vi "Generate Mass Spreadsheet Data.vi"() -> ()   [LabVIEW 2010]
uses:
  Controls/Spreadsheet Commands.ctl
  <vilib>/measure/NI_MABase.lvlib
panel:
  out "F-format string":string[][](array[string])
  in  "Channel Names":string[](array[string])
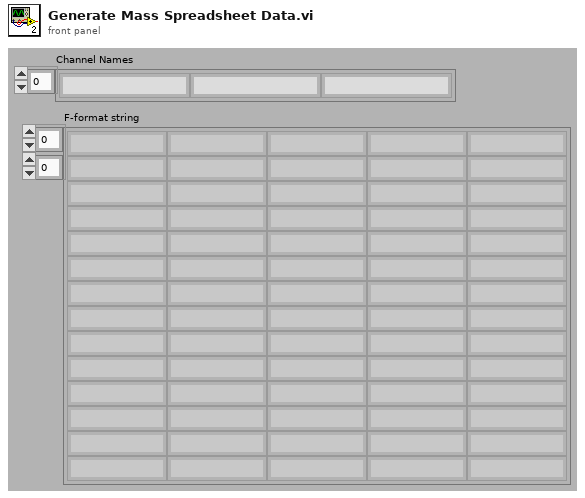
[diagram p1: front panel]
types:
  T1 = typedef "Spreadsheet Commands.ctl" = enum16{"Init", "Clear", "Add", "Mass Add", "Delete Row", "Format Colors", "Stop"}
  T2 = enum16{"Sine Wave", "Triangle Wave", "Square Wave", "Sawtooth Wave"}
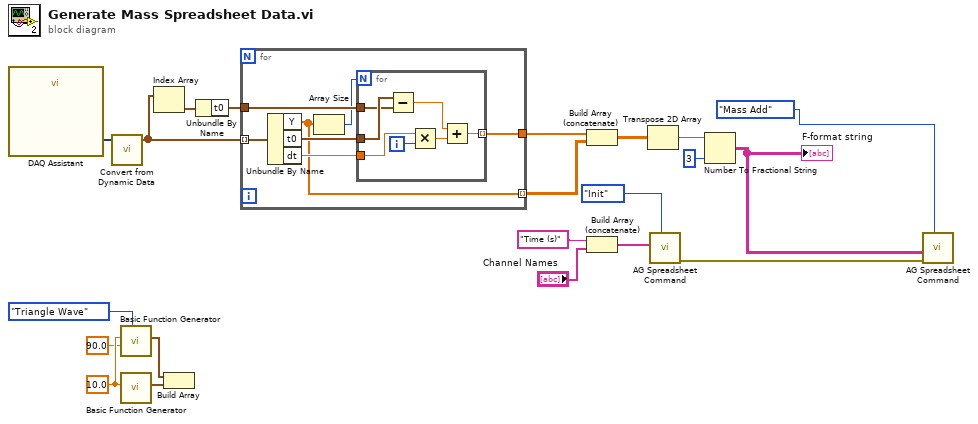
[diagram p0: block diagram]
diagram:
  w16 = 10.0 ("amplitude")
  n1 = call "DAQ Assistant"() -> ("data"=w11:dynamicdata)  [unwired: 17 in, 2 out]
  n2 = call "Convert from Dynamic Data"("Dynamic Data Type"=w11) -> ("Array of Waveform"=w7:waveform(dbl)[])  [unwired: 3 in]
  n3 = call <vilib>:"Basic Function Generator.vi"("signal type"=T2."Triangle Wave", "phase"=90.0, "amplitude"=w16) -> ("signal out"=w18:waveform(dbl))  [unwired: 6 in, 2 out]
  n4 = call <vilib>:"Basic Function Generator.vi"("amplitude"=w16) -> ("signal out"=w19:waveform(dbl))  [unwired: 8 in, 2 out]
  n5 = Index Array(array=w7) -> (element=w21:waveform(dbl))  [unwired: 1 in]
  n6 = Build Array(w18, w19) -> ()  [unwired: 1 out]
  n7 = Unbundle By Name(w21) -> ("t0"=w20:timestamp)
  n8 = for {
    tunnel: w7 -> [w28] mode=indexing
    tunnel: w20 -> [w27]
    tunnel: [w23] -> w14 mode=indexing
    tunnel: [w22] -> w13
    n9 = Unbundle By Name(w28) -> ("Y"=w23:dbl[], "t0"=w26:timestamp, "dt"=w25:dbl)
    n10 = Array Size(array=w23) -> (size(s)=w24:i32)
    n11 = for {
      N: w24 -> [_]
      tunnel: w27 -> [w34]
      tunnel: w26 -> [w35]
      tunnel: w25 -> [w31]
      tunnel: [w29] -> w22 mode=indexing
      i -> [w32]
      n12 = Subtract(x=w35, y=w34) -> (x-y=w33:dbl)
      n13 = Multiply(x=w31, y=w32) -> (x*y=w30:dbl)
      n14 = Add(x=w33, y=w30) -> (x+y=w29:dbl)
    }
  }
  n15 = Build Array (concatenate)(w13, w14) -> (w12:dbl[][])
  n16 = Build Array (concatenate)("Time (s)", "Channel Names") -> (w3:string[])
  n17 = Transpose 2D Array(2D array=w12) -> (transposed array=w10:dbl[][])
  n18 = call "AG Spreadsheet Command.vi"("Data"=w3, "Action (add)"=Spreadsheet_Commands."Init") -> ("error out"=w2:errorcluster)  [unwired: 8 in]
  n19 = Number To Fractional String(number=w10, precision (6)=i16 3) -> (F-format string=w6:string[][])  [unwired: 2 in]
  "F-format string" <- w6
  n20 = call "AG Spreadsheet Command.vi"("error in"=w2, "2D Data"=w6, "Action (add)"=Spreadsheet_Commands."Mass Add") -> ()  [unwired: 7 in, 1 out]
